vi "RSNRPZ Chans Meas Complete State.vi"(8 "error in (no error)":errorcluster, 11 "VISA session":refnum<visa-resource-name> caption="VISA resource name") -> (0 "error out":errorcluster, 2 "Measurement Completed":bool, 3 "dup VISA session":refnum<visa-resource-name> caption="VISA resource name")   [LabVIEW 2010]
doc: "This VI returns the summary status of measurements on all channels."
uses:
  rsnrpz_32.dll
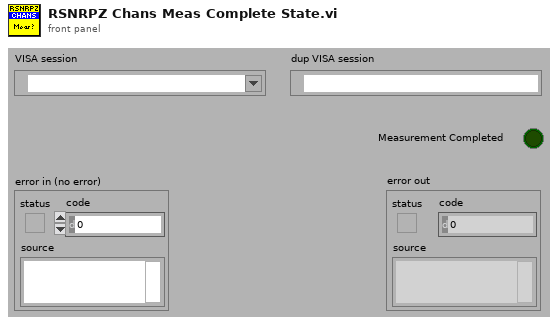
[diagram p1: front panel]
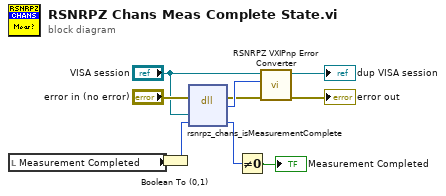
[diagram p0: block diagram]
diagram:
  n1 = local read "Measurement Completed"() -> (w9:bool)
  n2 = Boolean To (0,1)(Boolean=w9) -> (0, 1=w7:i16)
  n3 = dll-call lib="rsnrpz_32.dll" fn="rsnrpz_chans_isMeasurementComplete"(error in="error in (no error)", "VISA Session"="VISA session", "Measurement Completed"=w7) -> (error out=w5:errorcluster, "Status"=w10:i32, "Measurement Completed"=w8:u16)  [unwired: 3 in, 1 out]
  n4 = Not Equal To 0?(x=w8) -> (x != 0?=→"Measurement Completed":bool)
  n5 = call <instrlib>:"RSNRPZ VXIPnp Error Converter.vi"("error in"=w5, "VXIPnp error code"=w10, "VISA session"="VISA session") -> ("error out"=→"error out":errorcluster, "dup VISA session"=→"dup VISA session":refnum<visa-resource-name>)  [unwired: 7 in]
